vi "CSV.Load.vi"(8 "error in (no error)":errorcluster, 10 "Channel":string, 11 "selected path":path) -> (0 "error out":errorcluster, 2 "LUT":variant, 3 "path":path)   [LabVIEW 2019, in "OPC UA Client Addon System Explorer.lvlib"]
uses:
  OPC UA Client Addon System Explorer.lvlib
  <vilib>/Utility/miscctls.llb/LVStringsAndValuesArrayTypeDef_U32.ctl
  Types/Tag.TreeSettings.ctl
  <userlib>/_OpenG.lib/array/array.llb/Sort 2D Array (String)__ogtk.vi
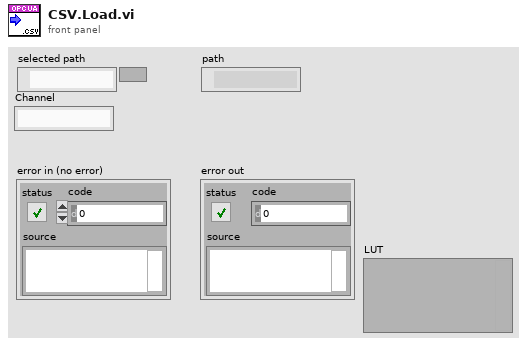
[diagram p1: front panel]
types:
  T1 = typedef "LVStringsAndValuesArrayTypeDef_U32.ctl" = cluster{"String":string, "Value":u32}[]
  T2 = enum16{"open", "replace", "create", "open or create", "replace or create", "replace or create with confirmation"}
  T3 = typedef "OPC UA Client Addon System Explorer.lvlib/Tag.TreeSettings.ctl" = cluster{"Settings":cluster{"name":string, "node type":enum32{"Other", "Folder", "Item/Property"}, "DataType":u32, "access":enum16{"Null", "Read", "Write", "Read&Write"}, "description":string}, "Array Size":i32}
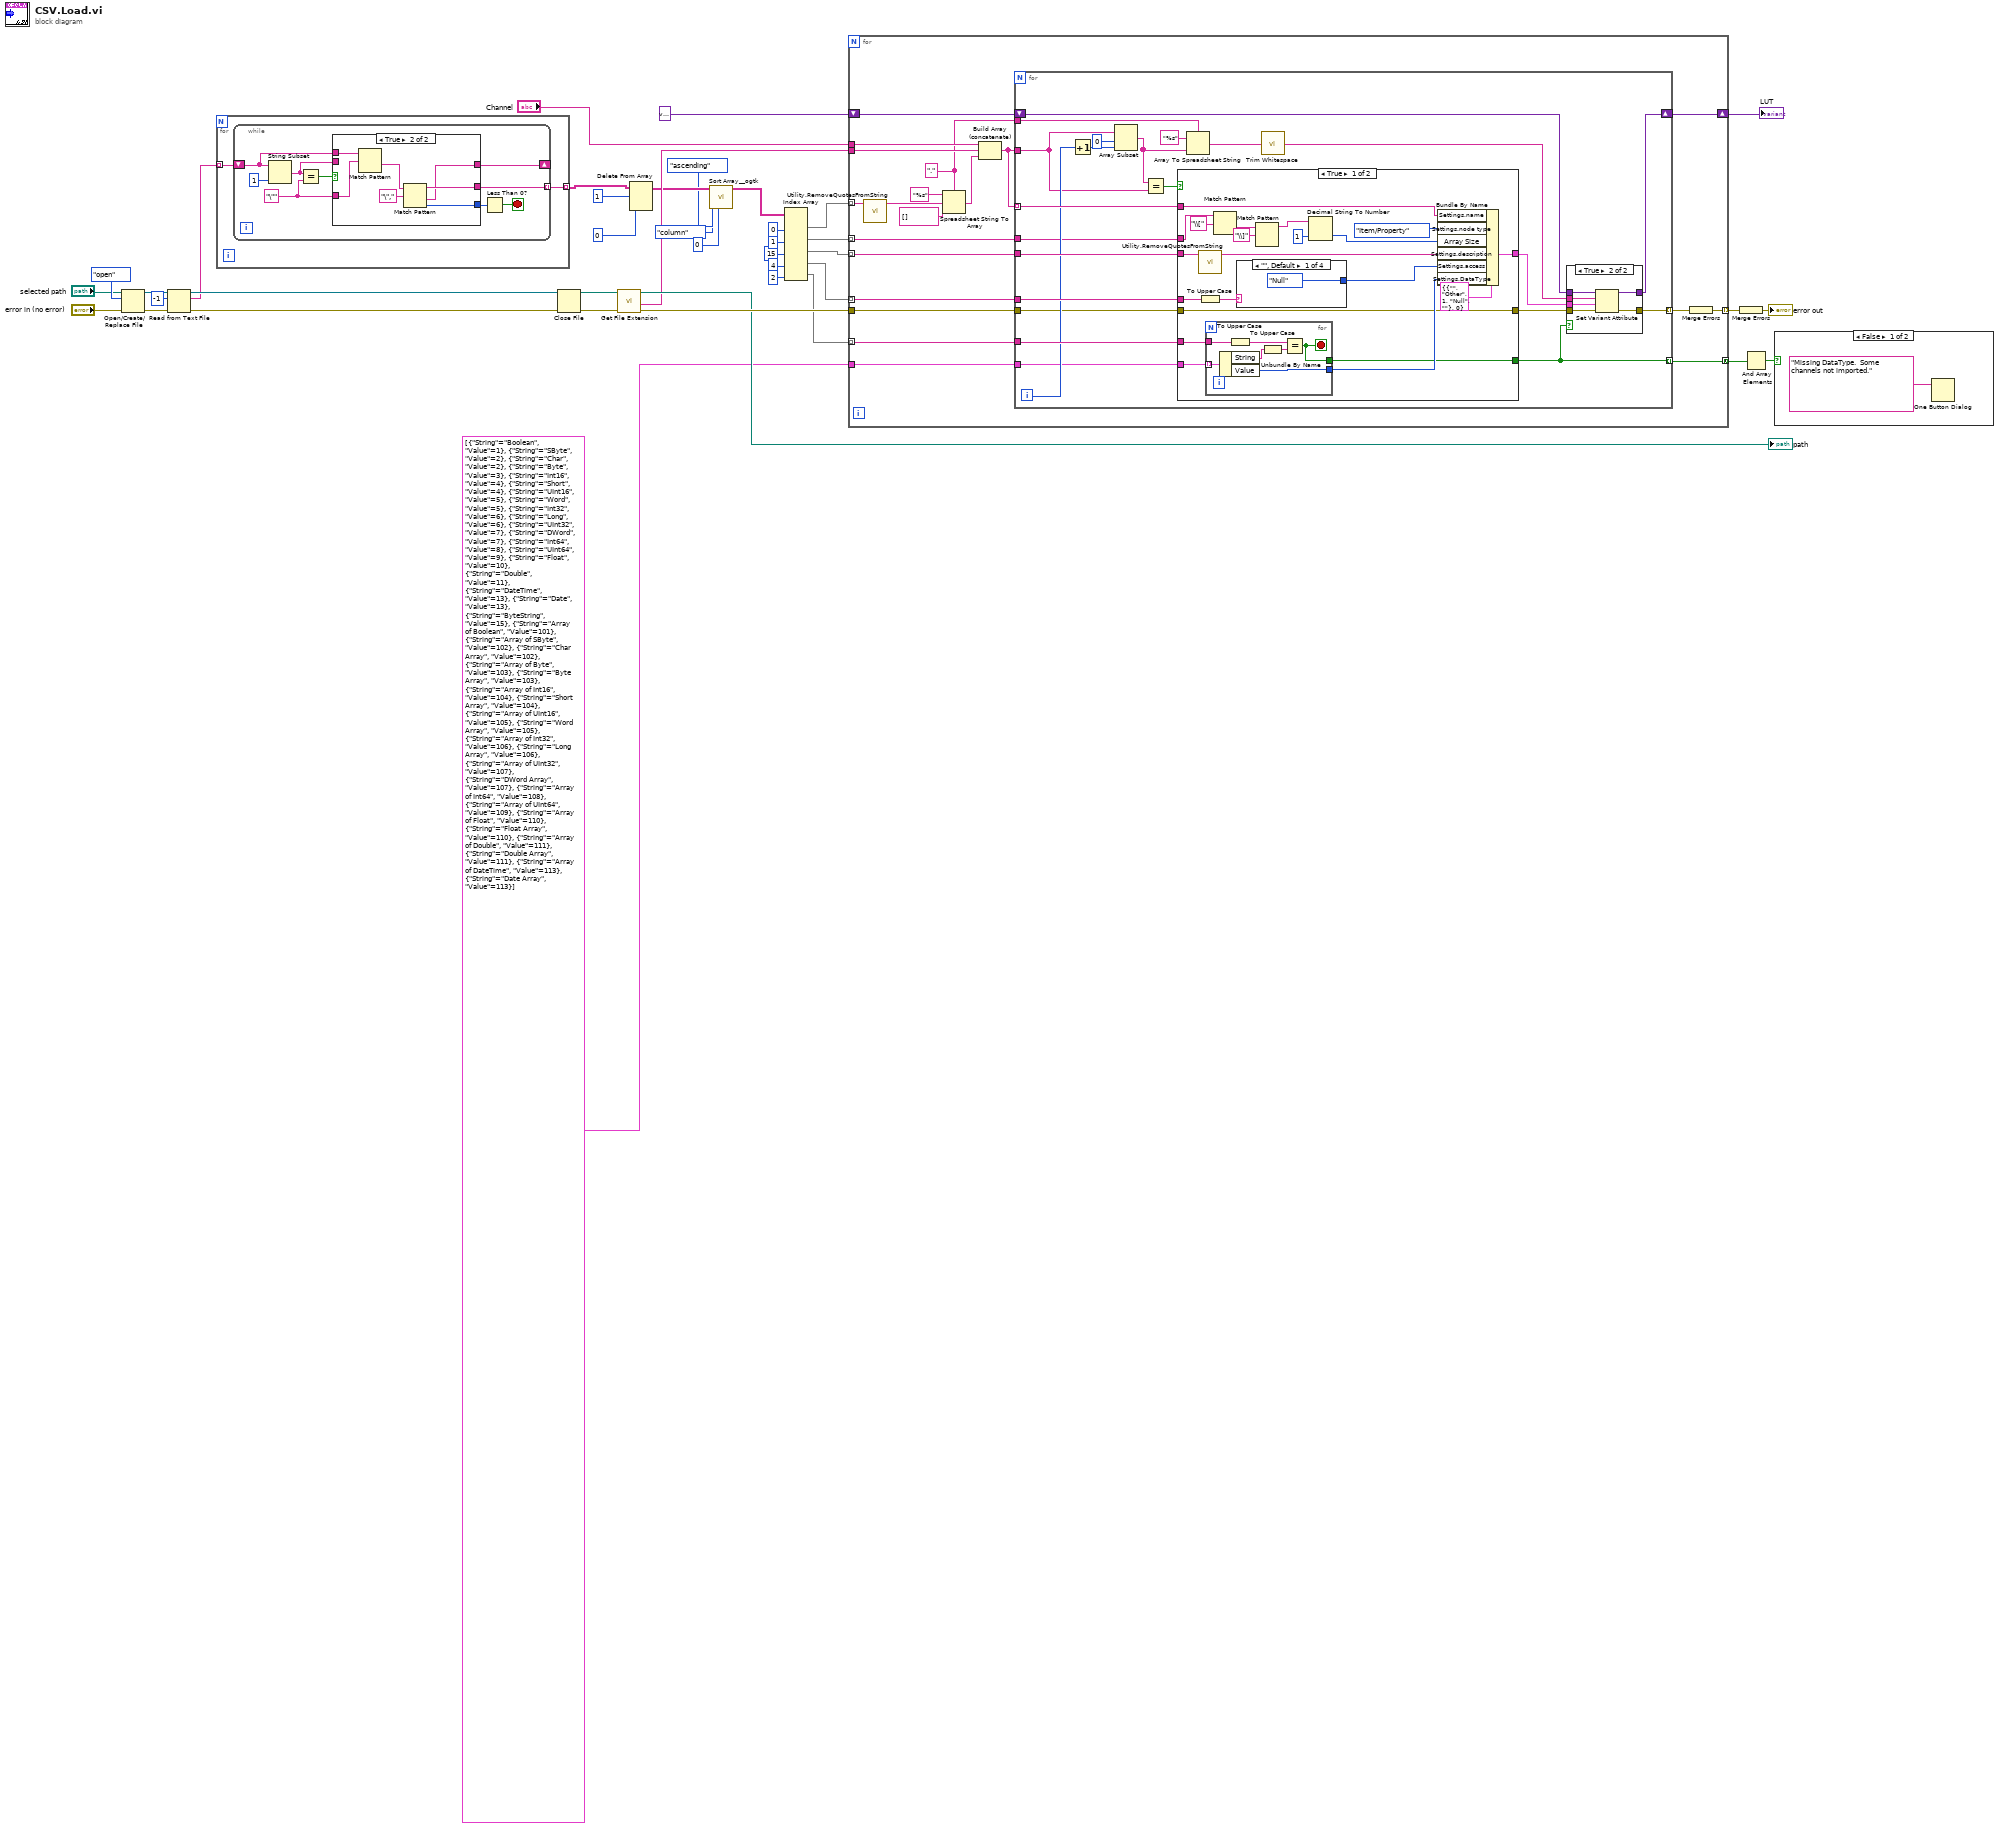
[diagram p0: block diagram]
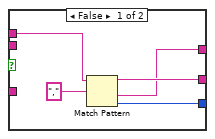
[diagram p2: hidden frame]
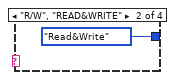
[diagram p5: hidden frame]
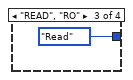
[diagram p6: hidden frame]
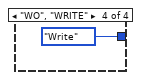
[diagram p7: hidden frame]
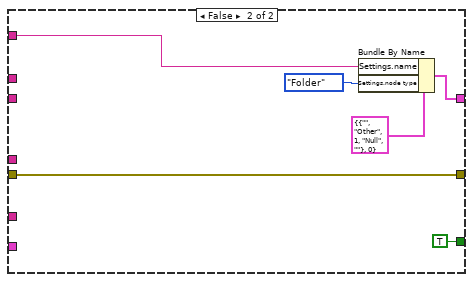
[diagram p8: hidden frame]
diagram:
  n1 = Open/Create/Replace File(file path (use dialog)="selected path", error in="error in (no error)", operation (0:open)=T2."open") -> (refnum out=w36:refnum<file>, error out=w33:errorcluster)  [unwired: 3 in, 1 out]
  n2 = Read from Text File(file (use dialog)=w36, count=-1, error in=w33) -> (refnum out=w35:refnum<file>, text=w3:string[], error out=w34:errorcluster)  [unwired: 1 in, 1 out]
  n3 = for {
    tunnel: w3 -> [w42] mode=indexing
    tunnel: [w41] -> w2 mode=indexing
    n4 = while {
      shift-right: [w44] -> _
      shift-left: w42 -> [w48]
      tunnel: [w45] -> w41 mode=indexing
      stop <- w47 stop-if-true
      w50 = "\"" ("regular expression")
      n5 = String Subset(string=w48, length (rest)=1 ("length (rest)")) -> (substring=w43:string)  [unwired: 1 in]
      n6 = Equal?(x=w43, y=w50) -> (x = y?=w49:bool)
      n7 = case shown="True" w49 {
        tunnel: w48 -> [w55 w58]
        tunnel: w50 -> [_ w59]
        tunnel: [w52 w62] -> w46
        tunnel: [w54 w61] -> w45
        tunnel: [w53 w60] -> w44
        tunnel: w43 -> [_ _]
        frame False {
          n8 = Match Pattern(string=w55, regular expression=",") -> (before substring=w54:string, after substring=w53:string, offset past match=w52:i32)  [unwired: 1 in, 1 out]
        }
        frame True {
          n9 = Match Pattern(string=w58, regular expression=w59) -> (after substring=w57:string)  [unwired: 1 in, 3 out]
          n10 = Match Pattern(string=w57, regular expression="\",") -> (before substring=w61:string, after substring=w60:string, offset past match=w62:i32)  [unwired: 1 in, 1 out]
        }
      }
      n11 = Less Than 0?(x=w46) -> (x < 0?=w47:bool)
    }
  }
  n12 = Close File(refnum=w35, error in=w34) -> (path=w25:path, error out=w27:errorcluster)
  n13 = call <vilib>:"Get File Extension.vi"("error in (no error)"=w27, "file"=w25) -> ("error out"=w26:errorcluster, "filename without extension"=w22:string, "dup file"=→"path":path)  [unwired: 5 in, 2 out]
  n14 = Delete From Array(array=w2, length=1, index (row)=0) -> (array with subset deleted=w18:string[][])  [unwired: 1 in, 1 out]
  n15 = call-poly <userlib>:"Sort Array__ogtk.vi"("Column/Row to Sort By"=u32 0, "Sort By in"=enum16{"row", "column"}."column", "Order"=enum16{"ascending", "descending"}."ascending", "Array in"=w18) -> ("Sorted Array out"=w17:string[][])  [unwired: 4 in, 3 out]
  n16 = Index Array(array=w17, index (col) #1=0 ("disabled index (col)"), index (col) #2=1 ("index (col)"), index (col) #3=15 ("index (col)"), index (col) #4=4 ("index (col)"), index (col) #5=2 ("index (col)")) -> (element #1=w31:string[], element #2=w6:string[], element #3=w8:string[], element #4=w10:string[], element #5=w12:string[])  [unwired: 5 in]
  n17 = for {
    tunnel: w12 -> [w81] mode=indexing
    tunnel: w10 -> [w82] mode=indexing
    tunnel: w8 -> [w83] mode=indexing
    tunnel: w31 -> [w68] mode=indexing
    shift-right: [w77] -> w21
    shift-left: variant ("variant") -> [w79]
    tunnel: "Channel" -> [w80]
    tunnel: w22 -> [w75]
    tunnel: T1 [{"String"="Boolean", "Value"=1}, {"String"="SByte", "Value"=2}, {"String"="Char", "Value"=2}, {"String"="Byte", "Value"=3}, {"String"="Int16", "Value"=4}, {"String"="Short", "Value"=4}, {"String"="UInt16", "Value"=5}, {"String"="Word", "Value"=5}, {"String"="Int32", "Value"=6}, {"String"="Long", "Value"=6}, {"String"="UInt32", "Value"=7}, {"String"="DWord", "Value"=7}, {"String"="Int64", "Value"=8}, {"String"="UInt64", "Value"=9}, {"String"="Float", "Value"=10}, {"String"="Double", "Value"=11}, {"String"="DateTime", "Value"=13}, {"String"="Date", "Value"=13}, {"String"="ByteString", "Value"=15}, {"String"="Array of Boolean", "Value"=101}, {"String"="Array of SByte", "Value"=102}, {"String"="Char Array", "Value"=102}, {"String"="Array of Byte", "Value"=103}, {"String"="Byte Array", "Value"=103}, {"String"="Array of Int16", "Value"=104}, {"String"="Short Array", "Value"=104}, {"String"="Array of UInt16", "Value"=105}, {"String"="Word Array", "Value"=105}, {"String"="Array of Int32", "Value"=106}, {"String"="Long Array", "Value"=106}, {"String"="Array of UInt32", "Value"=107}, {"String"="DWord Array", "Value"=107}, {"String"="Array of Int64", "Value"=108}, {"String"="Array of UInt64", "Value"=109}, {"String"="Array of Float", "Value"=110}, {"String"="Float Array", "Value"=110}, {"String"="Array of Double", "Value"=111}, {"String"="Double Array", "Value"=111}, {"String"="Array of DateTime", "Value"=113}, {"String"="Date Array", "Value"=113}] ("Strings And Values []") -> [w69]
    tunnel: w6 -> [w66] mode=indexing
    tunnel: [w65] -> w5 mode=concatenating
    tunnel: w26 -> [w74]
    tunnel: [w64] -> w20 mode=indexing
    w71 = "." ("delimiter (Tab)")
    n18 = call "Utility.RemoveQuotesFromString.vi"("String in"=w68) -> ("String out"=w67:string)  [unwired: 10 in]
    n19 = Spreadsheet String To Array(delimiter (Tab)=w71, format string="%s" ("spreadsheet string"), spreadsheet string=w67, array type (2D Dbl)=string[] []) -> (array=w73:string[])
    n20 = Build Array (concatenate)(w80, w75, w73) -> (w78:string[])
    n21 = for {
      tunnel: w78 -> [w103] mode=indexing
      tunnel: w83 -> [w106]
      tunnel: w82 -> [w105]
      tunnel: w81 -> [w104]
      tunnel: w78 -> [w96]
      shift-right: [w94] -> w77
      shift-left: w79 -> [w98]
      tunnel: w71 -> [w91]
      tunnel: w69 -> [w89]
      tunnel: w66 -> [w85]
      tunnel: [w84] -> w65 mode=indexing
      tunnel: w74 -> [w87]
      tunnel: [w99] -> w76 mode=indexing
      i -> [w100]
      n22 = Increment(x=w100) -> (x+1=w101:i32)
      n23 = Array Subset(array=w96, index=0, length=w101) -> (w93:string[])
      n24 = Equal?(x=w93, y=w96) -> (x = y?=w95:bool)
      n25 = case shown="True" w95 {
        tunnel: w106 -> [w127 _]
        tunnel: w105 -> [w134 _]
        tunnel: w104 -> [w131 _]
        tunnel: w103 -> [w129 w151]
        tunnel: [w124 w150] -> w97
        tunnel: w89 -> [w128 _]
        tunnel: w87 -> [w126 w149]
        tunnel: [w126 w149] -> w86
        tunnel: w85 -> [w122 _]
        tunnel: [w115 TRUE] -> w84
        frame True {
          n26 = call "Utility.RemoveQuotesFromString.vi"("String in"=w127) -> ("String out"=w123:string)  [unwired: 10 in]
          n27 = To Upper Case(1:w134) -> (0:w132:string)
          n28 = for {
            tunnel: w128 -> [w142] mode=indexing
            tunnel: w131 -> [w140]
            tunnel: [w137] -> w130
            tunnel: [w136] -> w115
            stop <- w136 stop-if-true
            n29 = Unbundle By Name(w142) -> ("String"=w141:string, "Value"=w137:u32)
            n30 = To Upper Case(1:w140) -> (0:w139:string)
            n31 = To Upper Case(1:w141) -> (0:w138:string)
            n32 = Equal?(x=w139, y=w138) -> (x = y?=w136:bool)
          }
          n33 = Match Pattern(string=w122, regular expression="\\[") -> (after substring=w120:string)  [unwired: 1 in, 3 out]
          n34 = case shown="\"\", Default" w132 {
            tunnel: [enum16{"Null", "Read", "Write", "Read&Write"}."Null" ("access") enum16{"Null", "Read", "Write", "Read&Write"}."Read&Write" ("access") enum16{"Null", "Read", "Write", "Read&Write"}."Read" ("access") enum16{"Null", "Read", "Write", "Read&Write"}."Write" ("access")] -> w133
            frame "", Default {
            }
            frame "R/W", "READ&WRITE" {
            }
            frame "READ", "RO" {
            }
            frame "WO", "WRITE" {
            }
          }
          n35 = Match Pattern(string=w120, regular expression="\\]") -> (before substring=w118:string)  [unwired: 1 in, 3 out]
          n36 = Decimal String To Number(string=w118, default (0L)=1 ("default (0 I32)")) -> (number=w116:i32)  [unwired: 1 in, 1 out]
          n37 = Bundle By Name(cluster=T3 {"Settings"={"name"="", "node type"=enum."Other", "DataType"=1, "access"=enum."Null", "description"=""}, "Array Size"=0}, "Settings.name"=w129, "Settings.node type"=enum32{"Other", "Folder", "Item/Property"}."Item/Property" ("node type"), "Array Size"=w116, "Settings.description"=w123, "Settings.access"=w133, "Settings.DataType"=w130) -> (w124:T3)
        }
        frame False {
          n38 = Bundle By Name(cluster=T3 {"Settings"={"name"="", "node type"=enum."Other", "DataType"=1, "access"=enum."Null", "description"=""}, "Array Size"=0}, "Settings.name"=w151, "Settings.node type"=enum32{"Other", "Folder", "Item/Property"}."Folder" ("node type")) -> (w150:T3)
        }
      }
      n39 = Array To Spreadsheet String(delimiter (Tab)=w91, array=w93, 3:"%s" ("format string")) -> (spreadsheet string=w92:string)
      n40 = call <vilib>:"Trim Whitespace.vi"("string"=w92) -> ("trimmed string"=w88:string)  [unwired: 1 in]
      n41 = case shown="True" w84 {
        tunnel: [w108 w114] -> w99
        tunnel: w98 -> [w107 w113]
        tunnel: w97 -> [_ w112]
        tunnel: [w107 w111] -> w94
        tunnel: w88 -> [_ w110]
        tunnel: w86 -> [w108 w109]
        frame False {
        }
        frame True {
          n42 = Set Variant Attribute(Variant=w113, name=w110, value=w112, error in=w109) -> (Variant out=w111:variant, error out=w114:errorcluster)  [unwired: 1 out]
        }
      }
    }
    n43 = Merge Errors(w76) -> (w64:errorcluster)
  }
  "LUT" <- w21
  n44 = Merge Errors(w20) -> (→"error out":errorcluster)
  n45 = And Array Elements(Boolean array=w5) -> (logical AND=w4:bool)
  n46 = case shown="False" w4 {
    frame False {
      n47 = One Button Dialog(message="Missing DataType.  Some channels not imported.") -> ()  [unwired: 1 in, 1 out]
    }
    frame True {
    }
  }
